vi "Get File Names.vi"(0 "configuration file path":path) -> (1 "file names":string[](array[string]), 2 "check sum":i16[](array[numeric]))   [LabVIEW 2017]
uses:
  <vilib>/Utility/config.llb/Read Key (I32).vi
  <vilib>/Utility/config.llb/NI_LVConfig.lvlib
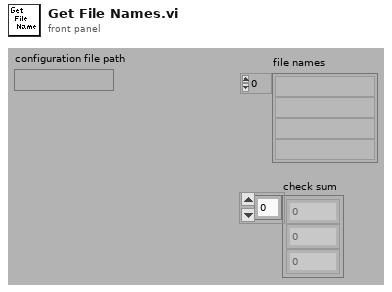
[diagram p1: front panel]
types:
  T1 = typedef "NI_LVConfig.lvlib/Config Data RefNum.ctl" = refnum<k1>
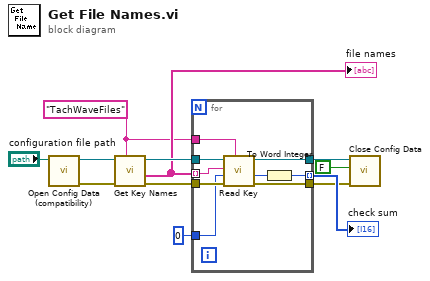
[diagram p0: block diagram]
diagram:
  w2 = "TachWaveFiles" ("section")
  n1 = call <vilib>:"Open Config Data (compatibility).vi"("configuration file path"="configuration file path") -> ("error out"=w6:errorcluster, "refnum"=w7:T1)  [unwired: 8 in, 1 out]
  n2 = call <vilib>:"Get Key Names.vi"("section"=w2, "error in (no error)"=w6, "refnum"=w7) -> ("error out"=w4:errorcluster, "key names"=w3:string[], "refnum out"=w5:T1)  [unwired: 5 in, 1 out]
  "file names" <- w3
  n3 = for {
    tunnel: w5 -> [w21]
    tunnel: w4 -> [w20]
    tunnel: w2 -> [w19]
    tunnel: w3 -> [w18] mode=indexing
    tunnel: 0 -> [w17]
    tunnel: [w15] -> w11 mode=indexing
    tunnel: [w14] -> w10
    tunnel: [w13] -> w9
    n4 = call-poly <vilib>:"Read Key.vi"("section"=w19, "error in (no error)"=w20, "default value"=w17, "key"=w18, "refnum"=w21) -> ("error out"=w13:errorcluster, "value"=w16:i32, "refnum out"=w14:T1)  [unwired: 3 in, 1 out]
    n5 = To Word Integer(number=w16) -> (16bit integer=w15:i16)
  }
  "check sum" <- w11
  n6 = call <vilib>:"Close Config Data.vi"("error in (no error)"=w9, "write file if changed (T)"=FALSE ("write configuration file? (T)"), "refnum"=w10) -> ()  [unwired: 7 in, 2 out]
